vi "Get Array of Elements.vi"(8 "Error In":errorcluster, 10 "Tag Name":string, 11 "Element In":refnum<k20>) -> (0 "Error Out":errorcluster, 1 "Nodes Values":string[](array[string]), 2 "Array Of Elements":refnum<k20>[](array[refnum]), 3 "Element Out":refnum<k20>)   [LabVIEW 2016, in "Tree Manager.lvclass"]
doc: "From th wired element return all child nodes with matching name."
uses:
  Tree Manager.lvclass
  <resource>/objmgr/DOMUserDefRef.rc
  <vilib>/xml/NI_XML.lvlib
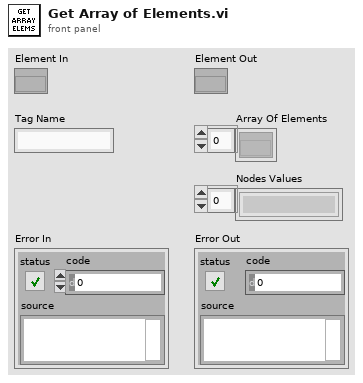
[diagram p1: front panel]
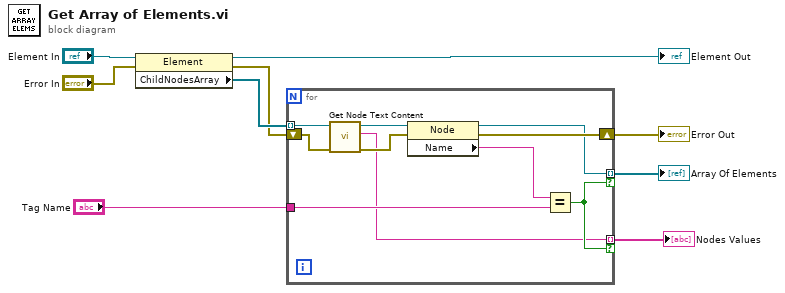
[diagram p0: block diagram]
diagram:
  n1 = property class="Element"(reference="Element In", error in="Error In") -> (reference out=→"Element Out":refnum<k20>, error out=w5:errorcluster, "ChildNodesArray"=w6:refnum<k20>[])
  n2 = for {
    tunnel: w6 -> [w14] mode=indexing
    shift-right: [w19] -> w3
    shift-left: w5 -> [w13]
    tunnel: [w18] -> w2 mode=indexing if=w15
    tunnel: "Tag Name" -> [w16]
    tunnel: [w10] -> w1 mode=indexing if=w15
    n3 = call <vilib>:"Get Node Text Content.vi"("error in (no error)"=w13, "node in"=w14) -> ("error out"=w12:errorcluster, "node text"=w10:string, "node out"=w11:refnum<k20>)  [unwired: 7 in]
    n4 = property class="Node"(reference=w11, error in=w12) -> (reference out=w18:refnum<k20>, error out=w19:errorcluster, "Name"=w17:string)
    n5 = Equal?(x=w17, y=w16) -> (x = y?=w15:bool)
  }
  "Array Of Elements" <- w2
  "Error Out" <- w3
  "Nodes Values" <- w1
